vi "Calculate_Hi-Tec_Demand.vi"(0 "Gas Line Name":string, 1 "Carrier Info":string, 2 "Flowrate":dbl=20.0 format="%.2f", 3 "Release temp (deg C)":dbl=20.0 format="%.2f", 4 "Mode":enum16{"Control Hi-Tec", "Check Hi-Tec Demands"}(ring), 5 "Atmos Pres (mbars)":dbl=1000.0 format="%.2f") -> (6 "Demand Voltage":dbl format="%.2f", 7 "Flowrate (kg/min)":dbl format="%.4f", 8 "Error messages":string)   [LabVIEW 2021]
uses:
  Anemometry/Anemometry Sub Vis/Globals/Gas_management_global.vi
panel:
  # "-Carrier 1 only\n-Carrier 2 only\n-Enter Ratio"
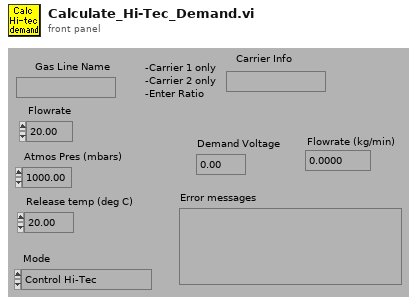
[diagram p1: front panel]
types:
  T1 = enum16{"Q(release) to Volts", "Volts to Q(release)"}
  T2 = typedef "Hi-Tec_calib.ctl" = cluster{"Ref temp (deg C)":dbl, "Ref Pres (mbars)":dbl, "Density at calib conditions":dbl, "Coefficients":dbl[]}
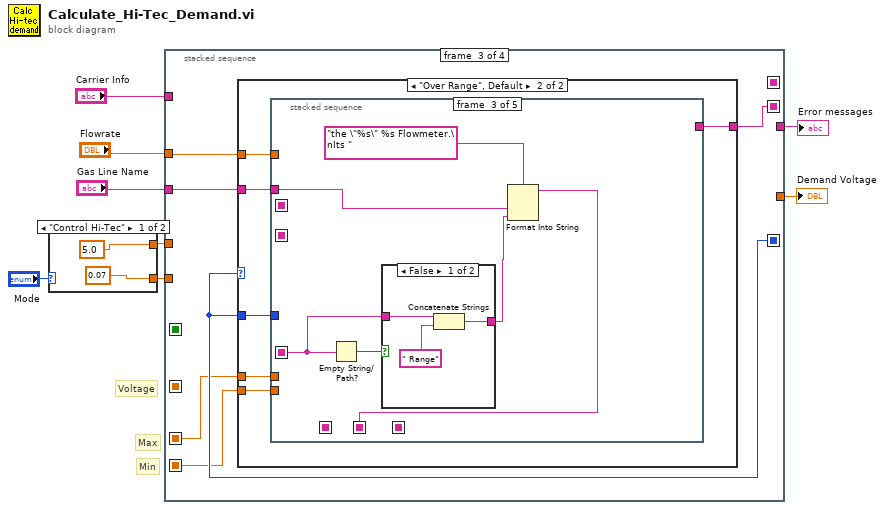
[diagram p0: block diagram]
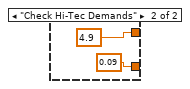
[diagram p2: hidden frame]
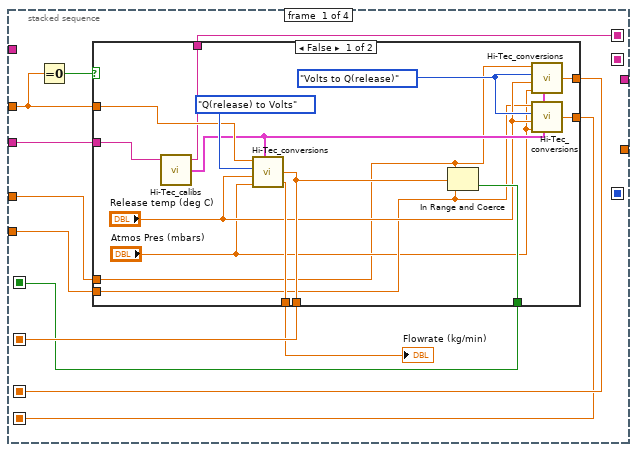
[diagram p3: hidden frame]
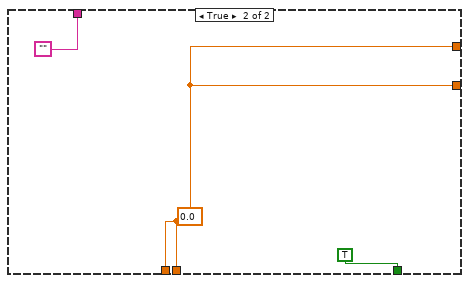
[diagram p4: hidden frame]
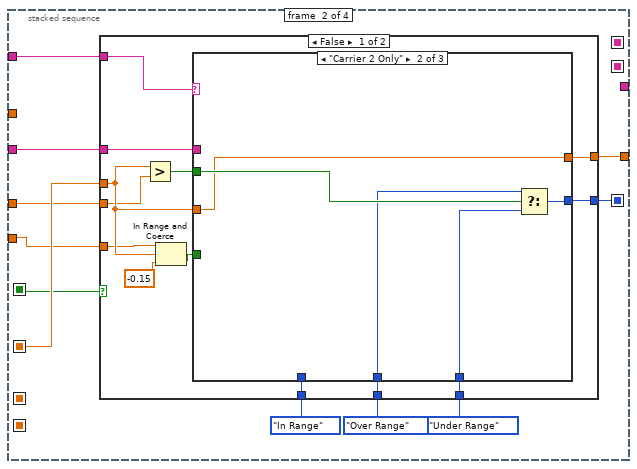
[diagram p5: hidden frame]
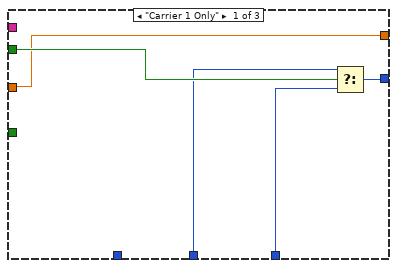
[diagram p6: hidden frame]
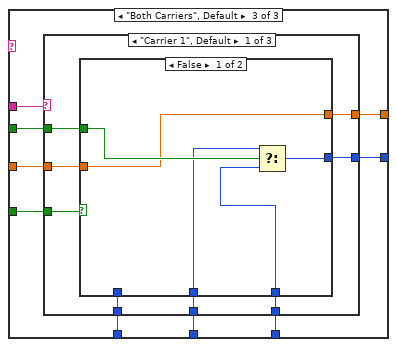
[diagram p7: hidden frame]
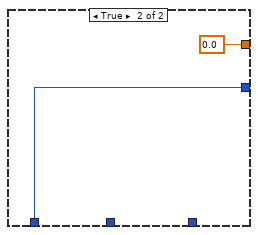
[diagram p8: hidden frame]
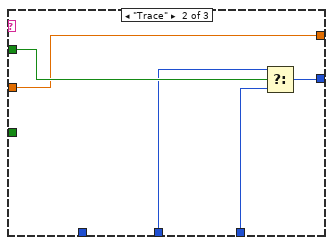
[diagram p9: hidden frame]
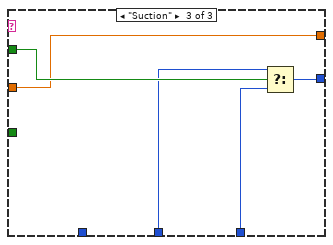
[diagram p10: hidden frame]
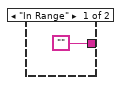
[diagram p12: hidden frame]
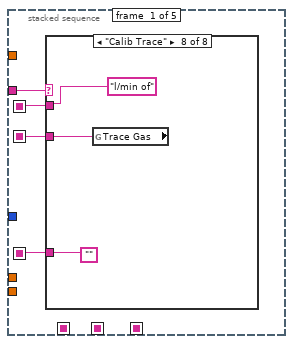
[diagram p13: hidden frame]
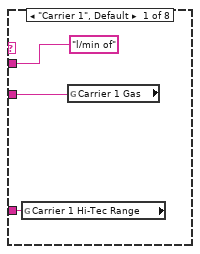
[diagram p14: hidden frame]
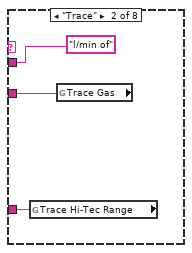
[diagram p15: hidden frame]
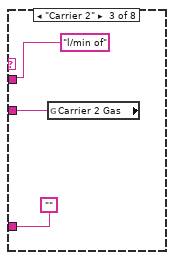
[diagram p16: hidden frame]
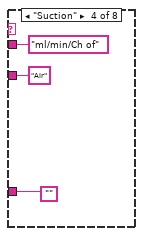
[diagram p17: hidden frame]
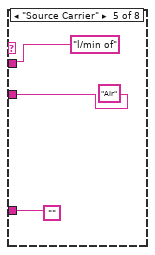
[diagram p18: hidden frame]
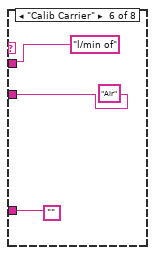
[diagram p19: hidden frame]
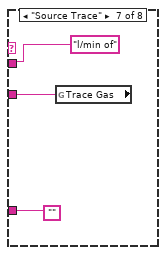
[diagram p20: hidden frame]
diagram:
  # "Min"
  # "Max"
  # "Voltage"
  n1 = case shown="\"Control Hi-Tec\"" "Mode" {
    tunnel: [5.0 ("y") 4.9 ("y")] -> w2
    tunnel: [0.07 ("lo") 0.09 ("lo")] -> w1
    frame "Control Hi-Tec" {
    }
    frame "Check Hi-Tec Demands" {
    }
  }
  n2 = stacked-sequence {
    seq-local: [w22 _ _ _] -> [_ w51 _ _]
    seq-local: [w19 _ _ _] -> [_ w50 _ _]
    seq-local: [_ w47 _ _] -> [_ _ w116 _]
    seq-local: [w17 _ _ _] -> [_ _ w114 _]
    seq-local: [w16 _ _ _] -> [_ _ w113 _]
    seq-local: [w13 _ _ _] -> [_ _ _ w192]
    seq-local: [_ _ w112 _] -> [_ _ _ w191]
    tunnel: "Gas Line Name" -> [w23 w49 w117 _]
    tunnel: "Flowrate" -> [w21 _ w115 _]
    tunnel: [_ w52 _ _] -> w6
    tunnel: [_ _ _ w190] -> w5
    tunnel: "Carrier Info" -> [_ w44 _ _]
    tunnel: w2 -> [w15 w43 _ _]
    tunnel: w1 -> [w14 w42 _ _]
    frame #0 {
      n3 = Equal To 0?(x=w21) -> (x = 0?=w20:bool)
      n4 = case shown="False" w20 {
        tunnel: w23 -> [w37 _]
        tunnel: [w36 w40] -> w22
        tunnel: w21 -> [w35 _]
        tunnel: [w34 TRUE] -> w19
        tunnel: [w33 w40] -> w18
        tunnel: [w29 w40] -> w17
        tunnel: [w28 w40] -> w16
        tunnel: w15 -> [w25 _]
        tunnel: w14 -> [w27 _]
        tunnel: [w24 ""] -> w13
        frame False {
          w31 = T1."Volts to Q(release)" ("Conversion")
          n5 = call "Hi-Tec_calibs.vi"("Gas Line Name"=w37) -> ("Hi-Tec calib"=w32:T2, "Comments"=w24:string)  [unwired: 1 in, 2 out]
          n6 = call "Hi-Tec_conversions.vi"("Input"=w35, "Conversion"=T1."Q(release) to Volts", "Release temp (deg C)"="Release temp (deg C)", "Atmos Pres (mbars)"="Atmos Pres (mbars)", "Hi-Tec calib"=w32) -> ("Output"=w36:dbl, "Flowrate (kg/min)"=w33:dbl)  [unwired: 1 out]
          n7 = In Range and Coerce(upper limit=w25, x=w36, lower limit=w27) -> (In Range?=w34:bool)  [unwired: 1 out]
          n8 = call "Hi-Tec_conversions.vi"("Input"=w25, "Conversion"=w31, "Release temp (deg C)"="Release temp (deg C)", "Atmos Pres (mbars)"="Atmos Pres (mbars)", "Hi-Tec calib"=w32) -> ("Output"=w29:dbl)  [unwired: 2 out]
          n9 = call "Hi-Tec_conversions.vi"("Input"=w27, "Conversion"=w31, "Release temp (deg C)"="Release temp (deg C)", "Atmos Pres (mbars)"="Atmos Pres (mbars)", "Hi-Tec calib"=w32) -> ("Output"=w28:dbl)  [unwired: 2 out]
        }
        frame True {
          w40 = 0.0 ("Output")
        }
      }
      "Flowrate (kg/min)" <- w18
    }
    frame #1 {
      n10 = case shown="False" w50 {
        tunnel: [w57 w111] -> w52
        tunnel: w51 -> [w56 w111]
        tunnel: w49 -> [w65 _]
        tunnel: enum16{"In Range", "Over Range", "Under Range"}."In Range" -> [w62 w110]
        tunnel: [w61 w110] -> w47
        tunnel: enum16{"In Range", "Over Range", "Under Range"}."Over Range" -> [w59 _]
        tunnel: enum16{"In Range", "Over Range", "Under Range"}."Under Range" -> [w58 _]
        tunnel: w44 -> [w55 _]
        tunnel: w43 -> [w54 _]
        tunnel: w42 -> [w53 _]
        frame False {
          n11 = Greater?(x=w56, y=w54) -> (0:w60:bool)
          n12 = In Range and Coerce(upper limit=w53, x=w56, lower limit=-0.15 ("lo")) -> (In Range?=w63:bool)  [unwired: 1 out]
          n13 = case shown="\"Carrier 2 Only\"" w55 {
            tunnel: w65 -> [_ _ w84]
            tunnel: w63 -> [_ _ w83]
            tunnel: w62 -> [_ _ w82]
            tunnel: [w67 w72 w81] -> w61
            tunnel: w60 -> [w69 w74 w80]
            tunnel: w59 -> [w68 w73 w79]
            tunnel: w58 -> [w70 w75 w78]
            tunnel: [w66 w71 w77] -> w57
            tunnel: w56 -> [w66 w71 w76]
            frame "Carrier 1 Only" {
              n14 = Select(t=w68, s=w69, f=w70) -> (s? t:f=w67:enum16{"In Range", "Over Range", "Under Range"})
            }
            frame "Carrier 2 Only" {
              n15 = Select(t=w73, s=w74, f=w75) -> (s? t:f=w72:enum16{"In Range", "Over Range", "Under Range"})
            }
            frame "Both Carriers", Default {
              n16 = case shown="\"Carrier 1\", Default" w84 {
                tunnel: w83 -> [w92 _ _]
                tunnel: w82 -> [w91 _ _]
                tunnel: [w90 w103 w108] -> w81
                tunnel: w80 -> [w89 w104 w109]
                tunnel: w79 -> [w88 w102 w107]
                tunnel: w78 -> [w87 w101 w106]
                tunnel: [w86 w100 w105] -> w77
                tunnel: w76 -> [w85 w100 w105]
                frame "Carrier 1", Default {
                  n17 = case shown="False" w92 {
                    tunnel: w91 -> [_ w99]
                    tunnel: [w94 w99] -> w90
                    tunnel: w89 -> [w97 _]
                    tunnel: w88 -> [w96 _]
                    tunnel: w87 -> [w95 _]
                    tunnel: [w93 0.0 ("y")] -> w86
                    tunnel: w85 -> [w93 _]
                    frame False {
                      n18 = Select(t=w96, s=w97, f=w95) -> (s? t:f=w94:enum16{"In Range", "Over Range", "Under Range"})
                    }
                    frame True {
                    }
                  }
                }
                frame "Trace" {
                  n19 = Select(t=w102, s=w104, f=w101) -> (s? t:f=w103:enum16{"In Range", "Over Range", "Under Range"})
                }
                frame "Suction" {
                  n20 = Select(t=w107, s=w109, f=w106) -> (s? t:f=w108:enum16{"In Range", "Over Range", "Under Range"})
                }
              }
            }
          }
        }
        frame True {
        }
      }
    }
    frame #2 {
      n21 = case shown="\"Over Range\", Default" w116 {
        tunnel: ["" w121] -> w112
        tunnel: w117 -> [_ w124]
        tunnel: w116 -> [_ w123]
        tunnel: w115 -> [_ w122]
        tunnel: w114 -> [_ w120]
        tunnel: w113 -> [_ w119]
        frame "In Range" {
        }
        frame "Over Range", Default {
          n22 = stacked-sequence {
            seq-local: [w127 _ _ _ _] -> [_ w154 _ _ _]
            seq-local: [w126 _ _ _ _] -> [_ _ w167 _ _]
            seq-local: [_ w157 _ _ _] -> [_ _ _ _ w189]
            seq-local: [w125 _ _ _ _] -> [_ w155 _ _ _]
            seq-local: [_ _ w163 _ _] -> [_ _ _ _ w188]
            seq-local: [_ _ _ w175 _] -> [_ _ _ _ w187]
            tunnel: w124 -> [w128 _ w166 _ _]
            tunnel: w123 -> [_ w159 _ w179 _]
            tunnel: w122 -> [_ w156 _ _ _]
            tunnel: [_ _ _ _ w186] -> w121
            tunnel: w120 -> [_ _ _ w178 _]
            tunnel: w119 -> [_ _ _ w173 _]
            frame #0 {
              n23 = case shown="\"Calib Trace\"" w128 {
                tunnel: [w131 w134 w137 "Air" ("Carrier 2 Gas") "Air" ("Carrier 2 Gas") "Air" ("Carrier 2 Gas") w149 w152] -> w127
                tunnel: [w130 w133 "" "" "" "" "" ""] -> w126
                tunnel: ["l/min of" "l/min of" "l/min of" "ml/min/Ch of" "l/min of" "l/min of" "l/min of" "l/min of"] -> w125
                frame "Carrier 1", Default {
                  n24 = global read "Gas_management_global.vi" "Carrier 1 Hi-Tec Range"() -> (w130:string)
                  n25 = global read "Gas_management_global.vi" "Carrier 1 Gas"() -> (w131:string)
                }
                frame "Trace" {
                  n26 = global read "Gas_management_global.vi" "Trace Hi-Tec Range"() -> (w133:string)
                  n27 = global read "Gas_management_global.vi" "Trace Gas"() -> (w134:string)
                }
                frame "Carrier 2" {
                  n28 = global read "Gas_management_global.vi" "Carrier 2 Gas"() -> (w137:string)
                }
                frame "Suction" {
                }
                frame "Source Carrier" {
                }
                frame "Calib Carrier" {
                }
                frame "Source Trace" {
                  n29 = global read "Gas_management_global.vi" "Trace Gas"() -> (w149:string)
                }
                frame "Calib Trace" {
                  n30 = global read "Gas_management_global.vi" "Trace Gas"() -> (w152:string)
                }
              }
            }
            frame #1 {
              n31 = case shown="\"Under Range\"" w159 {
                tunnel: ["In" "Over" "Under"] -> w153
                frame "In Range" {
                }
                frame "Over Range" {
                }
                frame "Under Range" {
                }
              }
              n32 = Format Into String(format string="A flowrate of %.4f %s %s is an %s Demand for " ("Format String"), w156, w155, w154, w153) -> (resulting string=w157:string)  [unwired: 2 in, 1 out]
            }
            frame #2 {
              n33 = Empty String/Path?(string/path=w167) -> (empty?=w168:bool)
              n34 = case shown="False" w168 {
                tunnel: w167 -> [w171 _]
                tunnel: [w169 ""] -> w165
                frame False {
                  n35 = Concatenate Strings(w171, " Range" ("Substring")) -> (w169:string)
                }
                frame True {
                }
              }
              n36 = Format Into String(format string="the \"%s\" %s Flowmeter.\nIts ", w166, w165) -> (resulting string=w163:string)  [unwired: 2 in, 1 out]
            }
            frame #3 {
              n37 = case shown="\"Under Range\"" w179 {
                tunnel: [0.0 ("Output") w183 w184] -> w177
                tunnel: w178 -> [_ w183 _]
                tunnel: ["" "Maximum" "Minimum"] -> w176
                tunnel: w173 -> [_ _ w184]
                frame "In Range" {
                }
                frame "Over Range" {
                }
                frame "Under Range" {
                }
              }
              n38 = Format Into String(format string="%s possible flowrate is %.4f l/min.\n" ("Format String"), w176, w177) -> (resulting string=w175:string)  [unwired: 2 in, 1 out]
            }
            frame #4 {
              n39 = Concatenate Strings(w189, w188, w187) -> (w186:string)
            }
          }
        }
      }
    }
    frame #3 {
      n40 = Concatenate Strings(w192, w191) -> (w190:string)
    }
  }
  "Demand Voltage" <- w6
  "Error messages" <- w5
